vi "Read Hyperdrive class.vi"(8 "error in (no error)":errorcluster, 11 "Hyperspace_SpaceShip in":refnum<class "Hyperspace_SpaceShip.lvclass">) -> (0 "error out":errorcluster, 2 "Hyperdrive class":T1(ring), 3 "Hyperspace_SpaceShip out":refnum<class "Hyperspace_SpaceShip.lvclass">)   [LabVIEW 2021, in "Hyperspace_SpaceShip.lvclass"]
uses:
  Hyperspace_SpaceShip.lvclass
  Hyperspace_SpaceShip.lvclass/Hyperspace_SpaceShip.ctl
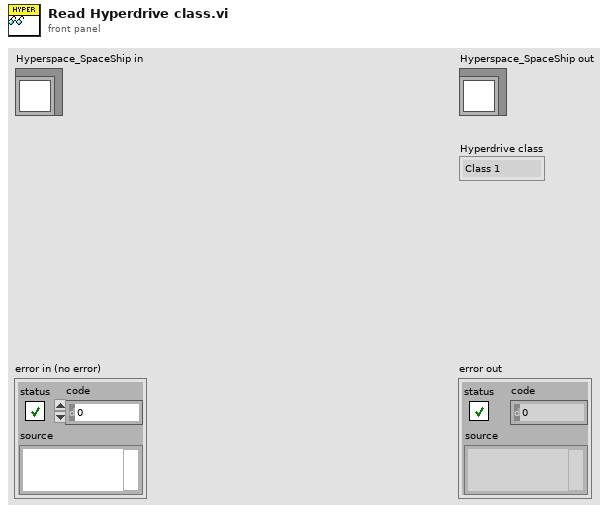
[diagram p1: front panel]
types:
  T1 = enum16{"Class 1", "Class 2", "Class 3", "Class 4"}
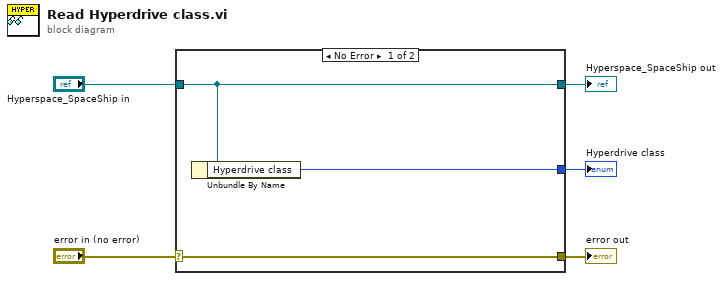
[diagram p0: block diagram]
diagram:
  n1 = case shown="No Error" "error in (no error)" {
    selector: "error in (no error)" -> [w8 w9]
    tunnel: [w8 w9] -> w4
    tunnel: [w7 w10] -> w2
    tunnel: "Hyperspace_SpaceShip in" -> [w7 w10]
    tunnel: [w6 _] -> w1
    frame No Error {
      n2 = Unbundle By Name(w7) -> ("Hyperdrive class"=w6:T1)
    }
    frame Error {
    }
  }
  "error out" <- w4
  "Hyperspace_SpaceShip out" <- w2
  "Hyperdrive class" <- w1
